vi "C8855-01_ReadLinesFromFile.vi"(2 "convert eol? (no:F)":bool, 3 "file path (dialog if empty)":path, 4 "number of lines (all:-1)":i32=-1, 7 "[pattern]":string caption="[パターン]", 8 "start of read offset (chars.:0 )":i32, 9 "[max characters per line]  (no limit:0)":i32) -> (0 "new file path (Not A Path if cancelled)":path, 1 "line string":string, 5 "mark after read (chars.)":i32, 6 "EOF?":bool)   [LabVIEW 2017]
doc: "Reads a specified number of lines from a byte stream file beginning at a specified character offset. The VI opens the file before reading from it and closes it afterwards."
panel:
  in  "prompt":string="Choose file to read."
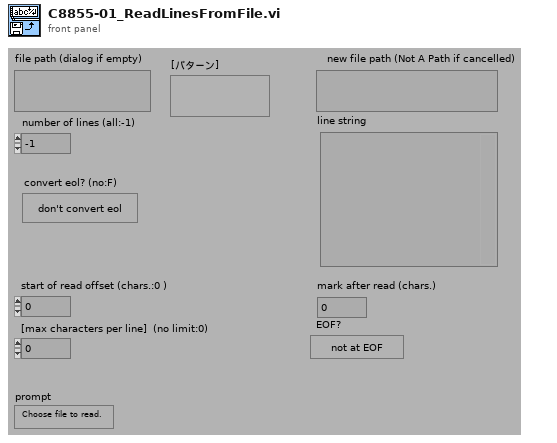
[diagram p1: front panel]
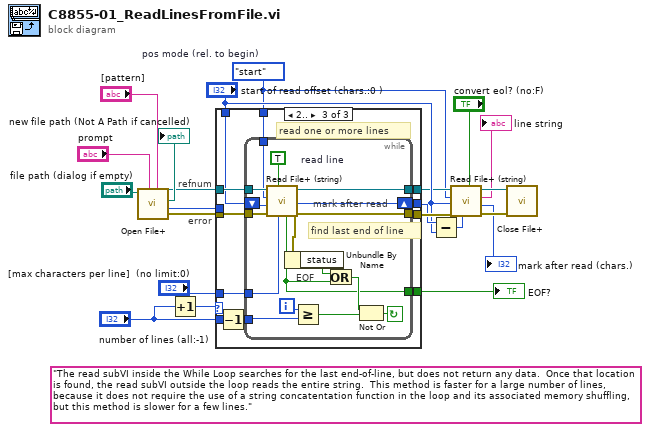
[diagram p0: block diagram]
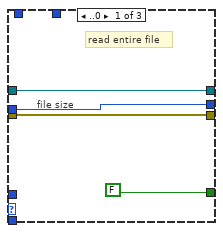
[diagram p2: hidden frame]
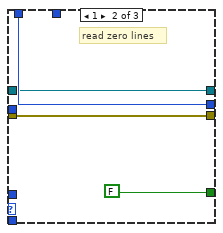
[diagram p3: hidden frame]
diagram:
  w3 = enum16{"start", "end", "current"}."start"  # pos mode (rel. to begin)
  (unwired) "The read subVI inside the While Loop searches for the last end-of-line, but does not return any data.  Once that location is found, the read subVI outside the loop reads the entire string.  This method is faster for a large number of lines, because it does not require the use of a string concatentation function in the loop and its associated memory shuffling, but this method is slower for a few lines."
  # "error"
  # "refnum"
  n1 = call <vilib>:"Open File+.vi"("[pattern]"="[pattern]", "prompt"="prompt", "file path (\" \")"="file path (dialog if empty)") -> ("error out"=w10:errorcluster, "file size (bytes)"=w7:i32, "file path"=→"new file path (Not A Path if cancelled)":path, "refnum"=w9:refnum<file>)  [unwired: 4 in, 1 out]
  n2 = Increment(x="number of lines (all:-1)") -> (x+1=w12:i32)
  n3 = case shown="2.." w12 {
    tunnel: [w26 w29 w41] -> w14
    tunnel: [w25 w30 w40] -> w13
    tunnel: "number of lines (all:-1)" -> [_ _ w39]
    tunnel: "[max characters per line]  (no limit:0)" -> [_ _ w38]
    tunnel: w10 -> [w26 w29 w37]
    tunnel: w9 -> [w24 w28 w36]
    tunnel: "start of read offset (chars.:0 )" -> [_ w30 w35]
    tunnel: w3 -> [_ _ w34]
    tunnel: w7 -> [w25 _ _]
    tunnel: [w24 w28 w33] -> w6
    tunnel: [FALSE FALSE w32] -> w5
    frame ..0 {
      # "file size"
      # "read entire file"
    }
    frame 1 {
      # "read zero lines"
    }
    frame 2.. {
      # "read one or more lines"
      n4 = Decrement(x=w39) -> (x-1=w31:i32)
      n5 = while {
        tunnel: [w43] -> w32
        tunnel: w34 -> [w48]
        tunnel: w37 -> [w50]
        tunnel: w38 -> [w51]
        tunnel: [w46] -> w41
        tunnel: w36 -> [w53]
        tunnel: [w54] -> w33
        tunnel: w31 -> [w42]
        shift-left: w35 -> [w55]
        shift-right: [w57] -> w40
        i -> [w56]
        stop <- w49 continue-if-true
        w45 = TRUE  # read line
        # "mark after read"
        # "find last end of line"
        # "EOF"
        n6 = call <vilib>:"Read File+ (string).vi"("count"=w51, "line mode (characters:F)"=w45, "error in (no error)"=w50, "pos offset (bytes:0)"=w55, "pos mode (rel. to current:2)"=w48, "refnum"=w53) -> ("error out"=w46:errorcluster, "mark after read (bytes)"=w57:i32, "dup refnum"=w54:refnum<file>, "EOF?"=w43:bool)  [unwired: 2 out]
        n7 = Unbundle By Name(w46) -> ("status"=w44:bool)
        n8 = Greater Or Equal?(x=w56, y=w42) -> (x >= y?=w52:bool)
        n9 = Or(x=w44, y=w43) -> (x .or. y?=w47:bool)
        n10 = Not Or(1:w52, 2:w47) -> (0:w49:bool)
      }
    }
  }
  "EOF?" <- w5
  n11 = Subtract(x=w13, y="start of read offset (chars.:0 )") -> (x-y=w19:i32)
  n12 = call <vilib>:"Read File+ (string).vi"("convert eol? (no:F)"="convert eol? (no:F)", "count"=w19, "error in (no error)"=w14, "pos offset (bytes:0)"="start of read offset (chars.:0 )", "pos mode (rel. to current:2)"=w3, "refnum"=w6) -> ("error out"=w20:errorcluster, "mark after read (bytes)"=→"mark after read (chars.)":i32, "string"=→"line string":string, "dup refnum"=w21:refnum<file>)  [unwired: 2 out]
  n13 = call <vilib>:"Close File+.vi"("error in (no error)"=w20, "refnum"=w21) -> ()  [unwired: 6 out]
